vi "TSLIN ChannelCount.vi"(0 "路径输入":path, 11 "错误输入（无错误）":errorcluster) -> (4 "路径输出":path, 15 "错误输出":errorcluster)   [LabVIEW 2013]
panel:
  out "LinCount":i32
  in  "使用通道数量":i32(ring)=1 items=["1通道"=1, "2通道"=2, "3通道"=3, "4通道"=4, "5通道"=5]
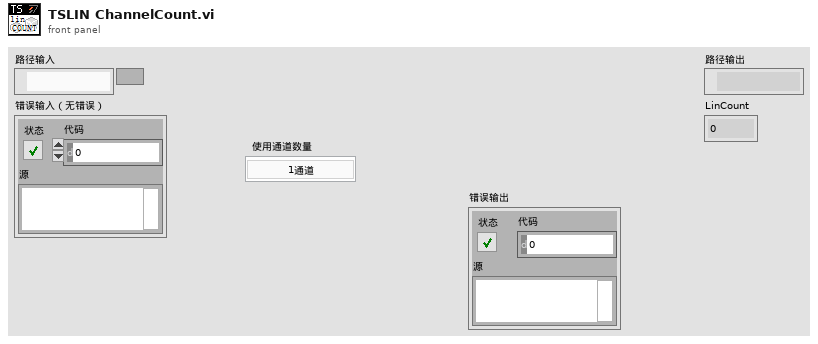
[diagram p1: front panel]
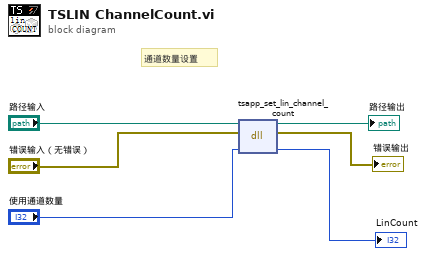
[diagram p0: block diagram]
diagram:
  # "通道数量设置"
  n1 = dll-call lib="PTH1@abs EDemo同星TSCAN_V1.4_20220301ConfigTSMaster.dll" fn="tsapp_set_lin_channel_count"(path in="路径输入", error in="错误输入（无错误）", "Aount"="使用通道数量") -> (path out=→"路径输出":path, error out=→"错误输出":errorcluster, "Aount"=→"LinCount":i32)  [unwired: 2 in]
